vi "for_v0_v10.vi"() -> ()   [LabVIEW 2010]
panel:
  in  "Start-Stop":bool
  in  "Iesire":bool
  out "Array":bool[](array[boolean])=[FALSE, TRUE, FALSE, FALSE, FALSE, FALSE, TRUE, FALSE]
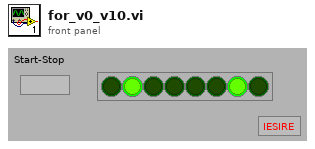
[diagram p1: front panel]
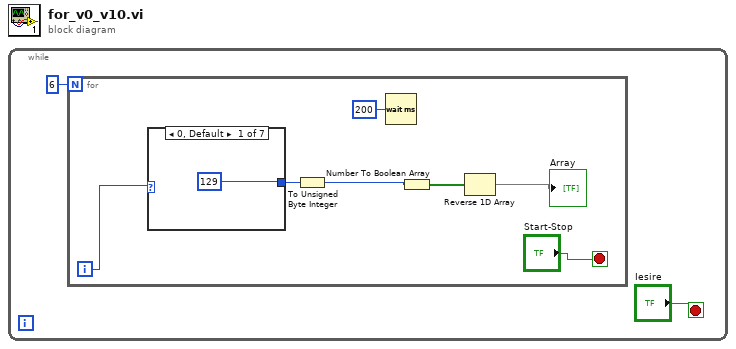
[diagram p0: block diagram]
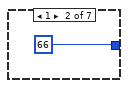
[diagram p2: hidden frame]
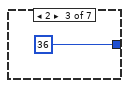
[diagram p3: hidden frame]
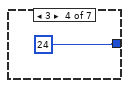
[diagram p4: hidden frame]
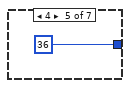
[diagram p5: hidden frame]
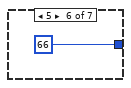
[diagram p6: hidden frame]
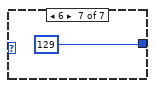
[diagram p7: hidden frame]
diagram:
  n1 = while {
    stop <- "Iesire" stop-if-true
    n2 = for {
      N: 6 -> [_]
      i -> [w5]
      stop <- "Start-Stop" stop-if-true
      n3 = case shown="0, Default" w5 {
        tunnel: [u8 129 u8 66 u8 36 u8 24 u8 36 u8 66 u8 129] -> w7
        frame 0, Default {
        }
        frame 1 {
        }
        frame 2 {
        }
        frame 3 {
        }
        frame 4 {
        }
        frame 5 {
        }
        frame 6 {
        }
      }
      n4 = To Unsigned Byte Integer(number=w7) -> (unsigned 8bit integer=w6:u8)
      n5 = Wait (ms)(milliseconds to wait=u32 200) -> ()  [unwired: 1 out]
      n6 = Number To Boolean Array(number=w6) -> (Boolean array=w9:bool[])
      n7 = Reverse 1D Array(array=w9) -> (reversed array=→"Array":bool[])
    }
  }
